vi "write_file_test_4loop.vi"() -> ()   [LabVIEW 2016]
uses:
  <vilib>/express/express signal manip/GetorSetDDTAttributes/Shared VIs/TimeType.ctl
  <vilib>/express/express signal manip/GetorSetDDTAttributes/Shared VIs/XDimension.ctl
  <vilib>/Utility/file.llb/Write Delimited Spreadsheet (DBL).vi
  <vilib>/express/express signal manip/GetorSetDDTAttributes/Shared VIs/XDimension Enum to String.vi
  <vilib>/express/express signal manip/GetorSetDDTAttributes/Shared VIs/TimeMode Enum to Boolean.vi
  <vilib>/express/express shared/transition.llb/Dynamic To Waveform Array.vi
  <vilib>/express/express signal manip/GetorSetDDTAttributes/Set DDT Attributes/SetT0.vi
  <vilib>/express/express signal manip/GetorSetDDTAttributes/Set DDT Attributes/sub Set StartTimeStamp.vi
  <vilib>/express/express shared/transition.llb/Waveform Array To Dynamic.vi
  <vilib>/express/express signal manip/GetorSetDDTAttributes/Set DDT Attributes/Set DDT Properties.xnode
  <vilib>/LabVIEW Interface for Arduino/LabVIEW Interface for Arduino.lvlib
  <vilib>/ptbypt/NI_PtbyPt.lvlib
  <vilib>/express/express signal manip/GetorSetDDTAttributes/Shared VIs/GetSetShared.lvlib
  <vilib>/express/express signal manip/GetorSetDDTAttributes/Set DDT Attributes/Set DDT Attributes.lvlib
panel:
  out "Voltage":dbl(knob) scale=0.0..5.0
  out "Numeric":i32
  in  "delimiter (\\t)":string="\t"
  in  "transpose? (no:F) 2":bool
  in  "append to file? (new file:F) 2":bool
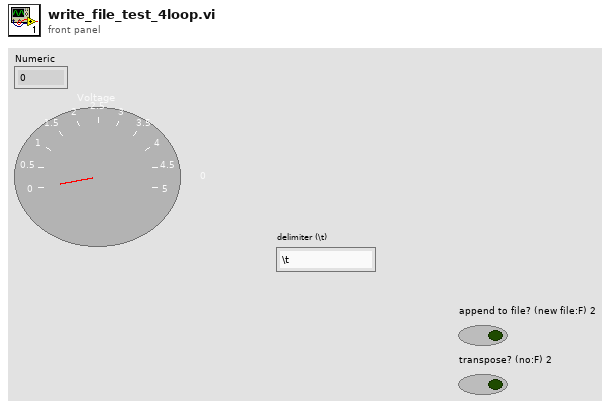
[diagram p1: front panel]
types:
  T1 = typedef "LabVIEW Interface for Arduino.lvlib/Arduino Resource.ctl" = cluster{"VISA resource":refnum<visa-resource-name>, "Board Type":T2, "Connection Type":enum8{"USB / Serial"}, "Bytes Per Packet (15)":u8}
  T2 = typedef "LabVIEW Interface for Arduino.lvlib/Board Type.ctl" = enum16{"Uno", "Dimuelanove w/Atmega 328", "Mega 2560"}
  T3 = typedef "GetSetShared.lvlib/XDimension.ctl" = enum16{"No Unit [-]", "Time [sec]", "Frequency [Hz]"}
  T4 = typedef "GetSetShared.lvlib/TimeType.ctl" = enum16{"Absolute", "Relative"}
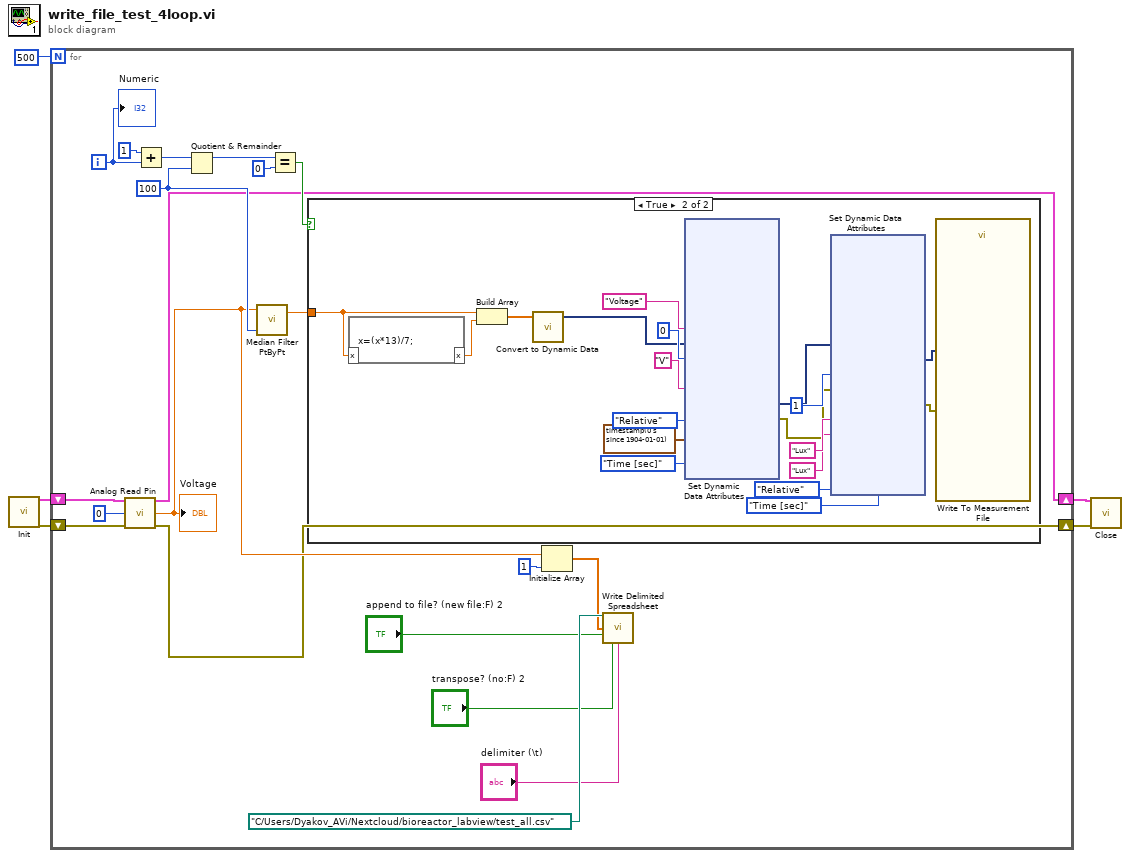
[diagram p0: block diagram]
diagram:
  n1 = call <vilib>:"Init.vi"() -> ("Arduino Resource"=w5:T1, "error out"=w4:errorcluster)  [unwired: 18 in]
  n2 = for {
    N: 500 -> [_]
    shift-right: [w7] -> w2
    shift-left: w5 -> [w14]
    shift-right: [w6] -> w1
    shift-left: w4 -> [w13]
    i -> [w11]
    w15 = 100 ("y")
    n3 = call <vilib>:"Analog Read Pin.vi"("Arduino Resource"=w14, "Analog Input Pin (0)"=u8 0, "error in"=w13) -> ("Arduino Resource"=w7:T1, "Voltage"=w10:dbl, "error out"=w6:errorcluster)  [unwired: 10 in]
    "Voltage" <- w10
    n4 = Add(x=1, y=w11) -> (x+y=w16:i32)
    n5 = Quotient & Remainder(x=w16, y=w15) -> (x-y*floor(x/y)=w19:i32)  [unwired: 1 out]
    n6 = call <vilib>:"Median Filter PtByPt.vi"("rank"=w15, "x"=w10) -> ("Filtered x"=w12:dbl)  [unwired: 2 in, 1 out]
    n7 = Equal?(x=w19, y=0) -> (x = y?=w8:bool)
    n8 = case shown="True" w8 {
      tunnel: w12 -> [_ w34]
      frame False {
      }
      frame True {
        n9 = formula code="x=(x*13)/7;"("x"=w34) -> ("x"=w35:dbl)
        n10 = Build Array(w34, w35) -> (w36:dbl[])
        n11 = call "Convert to Dynamic Data"("Array"=w36) -> ("Dynamic Data Type"=w33:dynamicdata)  [unwired: 3 in]
        n12 = xnode "Set Dynamic Data Attributes"("Signal Name"="Voltage", "Signals In"=w33, "Signal Index"=0, "Unit"="V", "Time Mode"=TimeType."Relative", "Start Timestamp"=timestamp(0 s since 1904-01-01), "X Dimension"=XDimension."Time [sec]") -> ("Signals Out"=w38:dynamicdata, "error out"=w29:errorcluster)  [unwired: 1 in]
        n13 = xnode "Set Dynamic Data Attributes"("Signals In"=w38, "Signal Index"=1, "error in"=w29, "Signal Name"="Lux", "Unit"="Lux", "Time Mode"=TimeType."Relative", "X Dimension"=XDimension."Time [sec]") -> ("Signals Out"=w37:dynamicdata, "error out"=w28:errorcluster)  [unwired: 1 in]
        n14 = call "Write To Measurement File"("Signals"=w37, "error in (no error)"=w28) -> ()  [unwired: 15 in, 3 out]
      }
    }
    n15 = Initialize Array(w10, 1 ("dimension size")) -> (w9:dbl[])
    n16 = call-poly <vilib>:"Write Delimited Spreadsheet.vi"("file path (dialog if empty)"=path "C:/Users/Dyakov_AVi/Nextcloud/bioreactor_labview/test_all.csv", "1D data"=w9, "append to file? (new file:F)"="append to file? (new file:F) 2", "transpose? (no:F)"="transpose? (no:F) 2", "delimiter (\\t)"="delimiter (\\t)") -> ()  [unwired: 9 in, 2 out]
    "Numeric" <- w11
  }
  n17 = call <vilib>:"Close.vi"("Arduino Resource"=w2, "error in"=w1) -> ()  [unwired: 13 in, 1 out]
